vi "Read Inv Sub (SubVI).vi"(11 "Array":string[](array[string])) -> (0 "Agua":i32, 1 "Galletas":i32, 2 "Refrescos":i32, 3 "Papas":i32)   [LabVIEW 2020, in "Productos.lvlib" / "Productos.lvclass"]
uses:
  Productos.lvclass
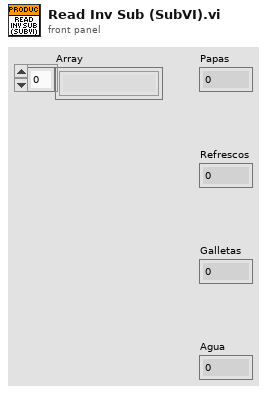
[diagram p1: front panel]
types:
  T1 = cluster{"Array[0]":string, "Array[1]":string, "Array[2]":string, "Array[3]":string, "Array[4]":string, "Array[5]":string, "Array[6]":string, "Array[7]":string, "Array[8]":string}
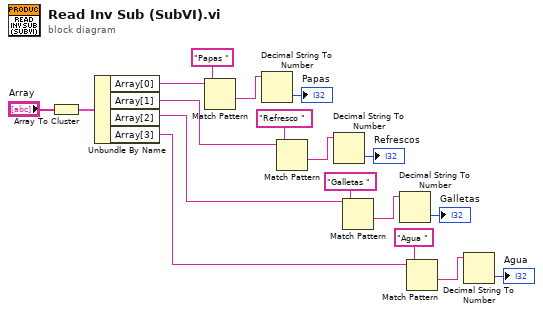
[diagram p0: block diagram]
diagram:
  n1 = Array To Cluster(array="Array") -> (cluster=w2:T1)
  n2 = Unbundle By Name(w2) -> ("Array[0]"=w3:string, "Array[1]"=w16:string, "Array[2]"=w17:string, "Array[3]"=w18:string)
  n3 = Match Pattern(string=w3, regular expression="Papas ") -> (after substring=w6:string)  [unwired: 1 in, 3 out]
  n4 = Decimal String To Number(string=w6) -> (number=→"Papas":i32)  [unwired: 2 in, 1 out]
  n5 = Match Pattern(string=w16, regular expression="Refresco ") -> (after substring=w7:string)  [unwired: 1 in, 3 out]
  n6 = Decimal String To Number(string=w7) -> (number=→"Refrescos":i32)  [unwired: 2 in, 1 out]
  n7 = Match Pattern(string=w17, regular expression="Galletas ") -> (after substring=w12:string)  [unwired: 1 in, 3 out]
  n8 = Decimal String To Number(string=w12) -> (number=→"Galletas":i32)  [unwired: 2 in, 1 out]
  n9 = Match Pattern(string=w18, regular expression="Agua ") -> (after substring=w13:string)  [unwired: 1 in, 3 out]
  n10 = Decimal String To Number(string=w13) -> (number=→"Agua":i32)  [unwired: 2 in, 1 out]
